vi "LOGFILE.vi"() -> ()   [LabVIEW 2020]
panel:
  in  "Output Enable (on)":bool=TRUE
  in  "Requested Bitrate kHz (1000)":u32=1000 max=50000
  out "Batch Length":i32
  in  "Byte Value (0x00)":u32 format="%.0x"
  in  "Byte Count (1)":u32=1 min=1
  in  "index":i32
  out "Actual Bitrate kHz":u32=1000
  in  "stop":bool
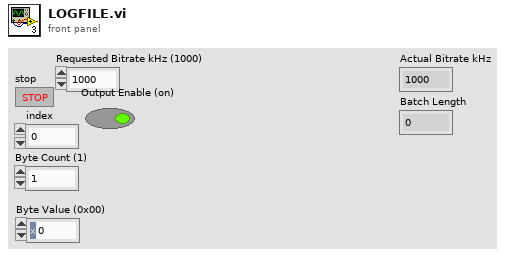
[diagram p1: front panel]
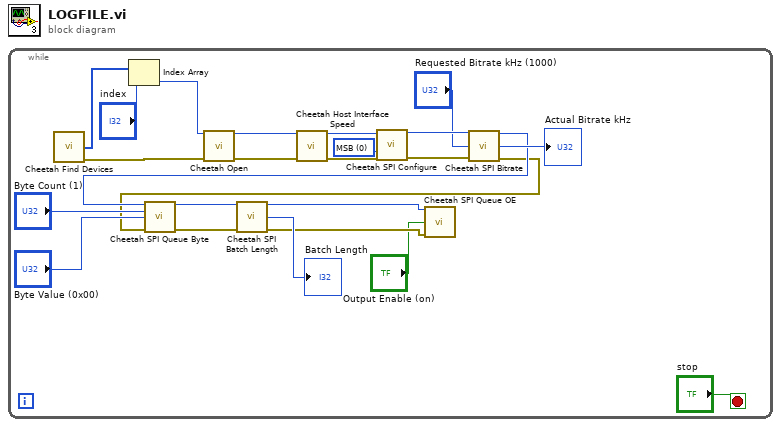
[diagram p0: block diagram]
diagram:
  n1 = while {
    stop <- "stop" stop-if-true
    w18 = 0 items=["MSB", "LSB"] ("Bitorder (0: MSB)")
    n2 = call <instrlib>:"Cheetah Find Devices.vi"() -> ("Ports"=w17:u16[], "error out"=w9:errorcluster)  [unwired: 13 in, 1 out]
    n3 = Index Array(array=w17, index="index") -> (element=w15:u16)
    n4 = call <instrlib>:"Cheetah Open.vi"("Port Number (0)"=w15, "error in (no error)"=w9) -> ("Cheetah Handle"=w13:i32, "error out"=w23:errorcluster)  [unwired: 12 in]
    n5 = call <instrlib>:"Cheetah Host Interface Speed.vi"("Cheetah Handle"=w13, "error in (no error)"=w23) -> ("dup Cheetah Handle"=w22:i32, "error out"=w21:errorcluster)  [unwired: 11 in, 1 out]
    n6 = call <instrlib>:"Cheetah SPI Configure.vi"("Cheetah Handle"=w22, "Bitorder (0: MSB)"=w18, "error in (no error)"=w21) -> ("dup Cheetah Handle"=w14:i32, "error out"=w20:errorcluster)  [unwired: 11 in]
    n7 = call <instrlib>:"Cheetah SPI Bitrate.vi"("Cheetah Handle"=w14, "Requested Bitrate kHz (1000)"="Requested Bitrate kHz (1000)", "error in (no error)"=w20) -> ("dup Cheetah Handle"=w12:i32, "Actual Bitrate kHz"=→"Actual Bitrate kHz":i32, "error out"=w8:errorcluster)  [unwired: 10 in]
    n8 = call <instrlib>:"Cheetah SPI Queue Byte.vi"("Cheetah Handle"=w12, "Byte Count (1)"="Byte Count (1)", "Byte Value (0x00)"="Byte Value (0x00)", "error in (no error)"=w8) -> ("dup Cheetah Handle"=w7:i32, "error out"=w6:errorcluster)  [unwired: 10 in]
    n9 = call <instrlib>:"Cheetah SPI Batch Length.vi"("Cheetah Handle"=w7, "error in (no error)"=w6) -> ("dup Cheetah Handle"=w3:i32, "Batch Length"=→"Batch Length":i32, "error out"=w2:errorcluster)  [unwired: 11 in]
    n10 = call <instrlib>:"Cheetah SPI Queue OE.vi"("Cheetah Handle"=w3, "Output Enable (on)"="Output Enable (on)", "error in (no error)"=w2) -> ()  [unwired: 11 in, 2 out]
  }
